vi "sv_Scale Factor for Change in Base Length Unit.vi"(5 "desired base units for length":i32(ring) items=["no change"=-1, "m"=0, "mm"=2, "microns"=3, "in"=1, "mils"=5], 7 "integration type":T1(ring), 8 "custom label in":string, 9 "engineering units in":T2 items=["custom..."=0, "V"=1, "A"=21, "C"=30, "pC"=31, "s"=32, "-"=29, "Pa"=2, "N"=20, "g"=3, "m/s^2"=4, "m/s"=5, "m"=6, "mm/s"=12, "mm"=13, "micron/s"=14, "micron"=15, "in/s^2"=7, "in/s"=8, "in"=9, "mil/s"=10, "mil"=11, "rad/s^2"=16, "rad/s"=17, "rad"=18, "deg/s^2"=26, "deg/s"=27, "deg"=28, "RPM"=22, "cycle/s^2"=23, "Hz"=24, "cycle"=25, "strain"=19], 10 "dB reference [EU] in":dbl) -> (0 "custom label out":string, 1 "engineering units out":T2 items=["custom..."=0, "V"=1, "A"=21, "C"=30, "pC"=31, "s"=32, "-"=29, "Pa"=2, "N"=20, "g"=3, "m/s^2"=4, "m/s"=5, "m"=6, "mm/s"=12, "mm"=13, "micron/s"=14, "micron"=15, "in/s^2"=7, "in/s"=8, "in"=9, "mil/s"=10, "mil"=11, "rad/s^2"=16, "rad/s"=17, "rad"=18, "deg/s^2"=26, "deg/s"=27, "deg"=28, "RPM"=22, "cycle/s^2"=23, "Hz"=24, "cycle"=25, "strain"=19], 2 "dB reference [EU] out":dbl, 3 "units scale factor":dbl)   [LabVIEW 2017]
uses:
  <vilib>/addons/_NISVFA/_Shared subVIs/Controls/svc_Engineering Units Text Ring.ctl
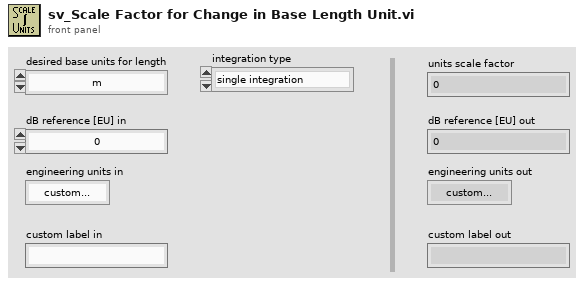
[diagram p1: front panel]
types:
  T1 = enum16{"single integration", "double integration"}
  T2 = typedef "svc_Engineering Units Text Ring.ctl" = u16
  T3 = enum16{"custom...", "V", "Pa", "g", "m/s^2", "m/s", "m", "in/s^2", "in/s", "in", "mil/s", "mil", "mm/s", "mm", "micron/s", "micron", "rad/s^2", "rad/s", "rad", "strain", "N", "A", "rpm", "cycle/s^2", "Hz", "cycle", "deg/s^2", "deg/s", "deg", "Undefined", "C", "pC"}
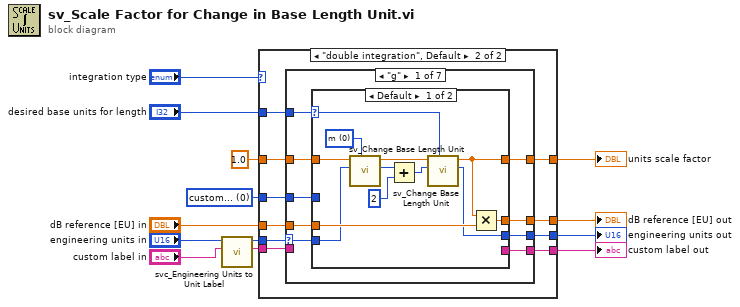
[diagram p0: block diagram]
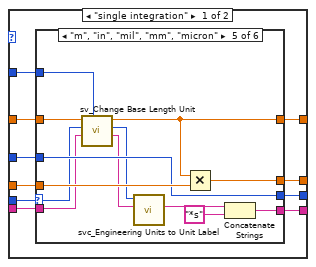
[diagram p2: hidden frame]
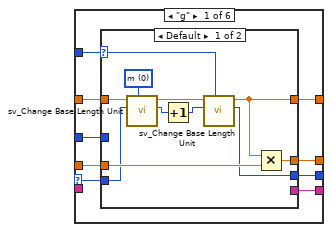
[diagram p3: hidden frame]
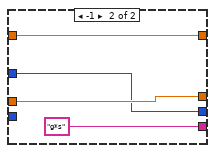
[diagram p4: hidden frame]
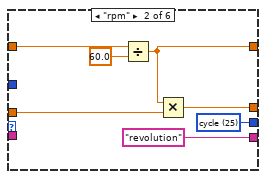
[diagram p5: hidden frame]
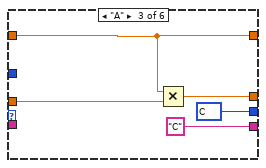
[diagram p6: hidden frame]
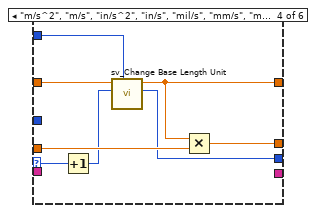
[diagram p7: hidden frame]
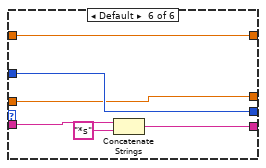
[diagram p8: hidden frame]
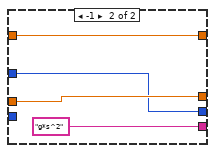
[diagram p9: hidden frame]
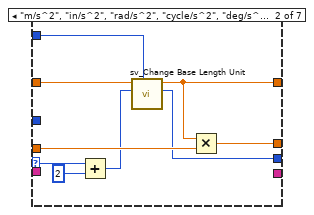
[diagram p10: hidden frame]
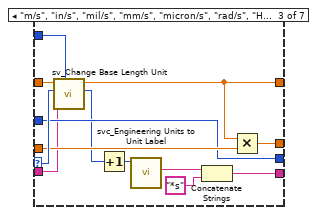
[diagram p11: hidden frame]
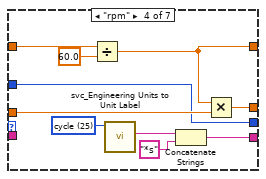
[diagram p12: hidden frame]
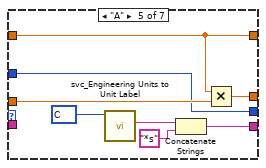
[diagram p13: hidden frame]
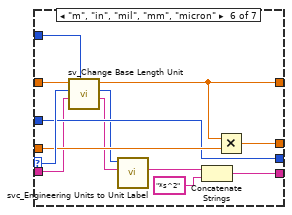
[diagram p14: hidden frame]
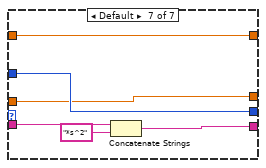
[diagram p15: hidden frame]
diagram:
  w10 = T2 0 items=["custom..."=0, "V"=1, "A"=21, "Pa"=2, "N"=20, "g"=3, "m/s^2"=4, "m/s"=5, "m"=6, "mm/s"=12, "mm"=13, "micron/s"=14, "micron"=15, "in/s^2"=7, "in/s"=8, "in"=9, "mil/s"=10, "mil"=11, "rad/s^2"=16, "rad/s"=17, "rad"=18, "m/m"=19] ("engineering units in")
  n1 = call <vilib>:"svc_Engineering Units to Unit Label.vi"("custom label"="custom label in", "engineering units"="engineering units in") -> ("unit label"=w8:string, "engineering units enum"=w2:T3)  [unwired: 8 in]
  n2 = case shown="\"double integration\", Default" "integration type" {
    tunnel: w2 -> [w23 w96]
    tunnel: [w22 w95] -> w6
    tunnel: 1.0 ("dB reference [EU]") -> [w21 w94]
    tunnel: "desired base units for length" -> [w19 w93]
    tunnel: "dB reference [EU] in" -> [w20 w92]
    tunnel: w8 -> [w18 w91]
    tunnel: [w17 w90] -> w9
    tunnel: [w16 w89] -> w11
    tunnel: [w14 w88] -> w12
    tunnel: w10 -> [w15 w87]
    frame "single integration" {
      n3 = case shown="\"m\", \"in\", \"mil\", \"mm\", \"micron\"" w23 {
        selector: w23 -> [w24 _ _ w62 w70 _]
        tunnel: [w31 w50 w55 w64 w77 w81] -> w22
        tunnel: w21 -> [w32 w54 w55 w67 w79 w81]
        tunnel: w20 -> [w30 w49 w57 w65 w76 w82]
        tunnel: w19 -> [w29 _ _ w66 w78 _]
        tunnel: w18 -> [_ _ _ _ w69 w85]
        tunnel: [w28 w48 w56 w63 w75 w82] -> w17
        tunnel: [w27 w52 w59 w60 w74 w84] -> w16
        tunnel: w15 -> [w25 _ _ _ w74 w84]
        tunnel: [w26 "revolution" ("Input Element") "C" ("Input Element") _ w73 w83] -> w14
        frame "g" {
          n4 = case shown="Default" w29 {
            selector: w29 -> [w35 _]
            tunnel: w32 -> [w39 w47]
            tunnel: [w34 w47] -> w31
            tunnel: w30 -> [w43 w46]
            tunnel: [w42 w46] -> w28
            tunnel: [w33 w44] -> w27
            tunnel: [_ "g*s" ("Input Element")] -> w26
            tunnel: w25 -> [_ w44]
            tunnel: w24 -> [w40 _]
            frame Default {
              w38 = 0 items=["no change"=-1, "m"=0, "mm"=2, "microns"=3, "in"=1, "mils"=5] ("desired base units for length")
              n5 = call <vilib>:"sv_Change Base Length Unit.vi"("desired base units for vibration"=w38, "engineering units in"=w40, "value in [EU]"=w39) -> ("engineering units out"=w41:T2, "value out [desired EU]"=w37:dbl)  [unwired: 4 in, 1 out]
              n6 = Increment(x=w41) -> (x+1=w36:T2)
              n7 = call <vilib>:"sv_Change Base Length Unit.vi"("desired base units for vibration"=w35, "engineering units in"=w36, "value in [EU]"=w37) -> ("engineering units out"=w33:T2, "value out [desired EU]"=w34:dbl)  [unwired: 4 in, 1 out]
              n8 = Multiply(x=w34, y=w43) -> (x*y=w42:dbl)
            }
            frame -1 {
            }
          }
        }
        frame "rpm" {
          w52 = T2 25 items=["custom..."=0, "V"=1, "A"=21, "Pa"=2, "N"=20, "g"=3, "m/s^2"=4, "m/s"=5, "m"=6, "mm/s"=12, "mm"=13, "micron/s"=14, "micron"=15, "in/s^2"=7, "in/s"=8, "in"=9, "mil/s"=10, "mil"=11, "rad/s^2"=16, "rad/s"=17, "rad"=18, "deg/s^2"=26, "deg/s"=27, "deg"=28, "RPM"=22, "cycle/s^2"=23, "Hz"=24, "cycle"=25, "strain"=19] ("engineering units in")
          n9 = Divide(x=w54, y=60.0) -> (x/y=w50:dbl)
          n10 = Multiply(x=w50, y=w49) -> (x*y=w48:dbl)
        }
        frame "A" {
          w59 = T2 30 items=["custom..."=0, "V"=1, "A"=21, "C"=30, "pC"=31, "s"=32, "-"=29, "Pa"=2, "N"=20, "g"=3, "m/s^2"=4, "m/s"=5, "m"=6, "mm/s"=12, "mm"=13, "micron/s"=14, "micron"=15, "in/s^2"=7, "in/s"=8, "in"=9, "mil/s"=10, "mil"=11, "rad/s^2"=16, "rad/s"=17, "rad"=18, "deg/s^2"=26, "deg/s"=27, "deg"=28, "RPM"=22, "cycle/s^2"=23, "Hz"=24, "cycle"=25, "strain"=19] ("engineering units in")
          n11 = Multiply(x=w55, y=w57) -> (x*y=w56:dbl)
        }
        frame "m/s^2", "m/s", "in/s^2", "in/s", "mil/s", "mm/s", "micron/s", "rad/s^2", "rad/s", "cycle/s^2", "Hz", "deg/s^2", "deg/s" {
          n12 = Increment(x=w62) -> (x+1=w61:T3)
          n13 = call <vilib>:"sv_Change Base Length Unit.vi"("desired base units for vibration"=w66, "engineering units in"=w61, "value in [EU]"=w67) -> ("engineering units out"=w60:T2, "value out [desired EU]"=w64:dbl)  [unwired: 4 in, 1 out]
          n14 = Multiply(x=w64, y=w65) -> (x*y=w63:dbl)
        }
        frame "m", "in", "mil", "mm", "micron" {
          n15 = call <vilib>:"sv_Change Base Length Unit.vi"("desired base units for vibration"=w78, "custom label in"=w69, "engineering units in"=w70, "value in [EU]"=w79) -> ("custom label out"=w68:string, "engineering units out"=w71:T2, "value out [desired EU]"=w77:dbl)  [unwired: 3 in]
          n16 = call <vilib>:"svc_Engineering Units to Unit Label.vi"("custom label"=w68, "engineering units"=w71) -> ("unit label"=w72:string)  [unwired: 8 in, 1 out]
          n17 = Multiply(x=w77, y=w76) -> (x*y=w75:dbl)
          n18 = Concatenate Strings(w72, "*s" ("Input Element")) -> (w73:string)
        }
        frame Default {
          n19 = Concatenate Strings(w85, "*s" ("Input Element")) -> (w83:string)
        }
      }
    }
    frame "double integration", Default {
      n20 = case shown="\"g\"" w96 {
        selector: w96 -> [w97 w124 w141 _ _ w172 _]
        tunnel: [w105 w129 w140 w145 w155 w171 w176] -> w95
        tunnel: w94 -> [w104 w130 w143 w147 w155 w174 w176]
        tunnel: w93 -> [w102 w127 w142 _ _ w173 _]
        tunnel: w92 -> [w103 w128 w139 w153 w161 w170 w175]
        tunnel: w91 -> [_ _ w131 _ _ w163 w179]
        tunnel: [w100 w126 w138 w152 w160 w169 w175] -> w90
        tunnel: [w101 w122 w137 w151 w159 w168 w177] -> w89
        tunnel: [w99 _ w136 w150 w158 w167 w178] -> w88
        tunnel: w87 -> [w98 _ w137 w151 w159 w168 w177]
        frame "g" {
          n21 = case shown="Default" w102 {
            selector: w102 -> [w115 _]
            tunnel: w104 -> [w109 w121]
            tunnel: [w116 w121] -> w105
            tunnel: w103 -> [w117 w120]
            tunnel: [w106 w118] -> w101
            tunnel: [w114 w120] -> w100
            tunnel: [_ "g*s^2" ("Input Element")] -> w99
            tunnel: w98 -> [_ w118]
            tunnel: w97 -> [w107 _]
            frame Default {
              w108 = 0 items=["no change"=-1, "m"=0, "mm"=2, "microns"=3, "in"=1, "mils"=5] ("desired base units for length")
              n22 = call <vilib>:"sv_Change Base Length Unit.vi"("desired base units for vibration"=w108, "engineering units in"=w107, "value in [EU]"=w109) -> ("engineering units out"=w112:T2, "value out [desired EU]"=w110:dbl)  [unwired: 4 in, 1 out]
              n23 = Add(x=w112, y=u16 2) -> (x+y=w111:T2)
              n24 = call <vilib>:"sv_Change Base Length Unit.vi"("desired base units for vibration"=w115, "engineering units in"=w111, "value in [EU]"=w110) -> ("engineering units out"=w106:T2, "value out [desired EU]"=w116:dbl)  [unwired: 4 in, 1 out]
              n25 = Multiply(x=w116, y=w117) -> (x*y=w114:dbl)
            }
            frame -1 {
            }
          }
        }
        frame "m/s^2", "in/s^2", "rad/s^2", "cycle/s^2", "deg/s^2" {
          n26 = Add(x=w124, y=u16 2) -> (x+y=w123:u16)
          n27 = call <vilib>:"sv_Change Base Length Unit.vi"("desired base units for vibration"=w127, "engineering units in"=w123, "value in [EU]"=w130) -> ("engineering units out"=w122:T2, "value out [desired EU]"=w129:dbl)  [unwired: 4 in, 1 out]
          n28 = Multiply(x=w129, y=w128) -> (x*y=w126:dbl)
        }
        frame "m/s", "in/s", "mil/s", "mm/s", "micron/s", "rad/s", "Hz", "deg/s" {
          n29 = call <vilib>:"sv_Change Base Length Unit.vi"("desired base units for vibration"=w142, "custom label in"=w131, "engineering units in"=w141, "value in [EU]"=w143) -> ("engineering units out"=w133:T2, "value out [desired EU]"=w140:dbl)  [unwired: 3 in, 1 out]
          n30 = Increment(x=w133) -> (x+1=w132:T2)
          n31 = call <vilib>:"svc_Engineering Units to Unit Label.vi"("engineering units"=w132) -> ("unit label"=w134:string)  [unwired: 9 in, 1 out]
          n32 = Concatenate Strings(w134, "*s" ("custom label")) -> (w136:string)
          n33 = Multiply(x=w140, y=w139) -> (x*y=w138:dbl)
        }
        frame "rpm" {
          w144 = T2 25 items=["custom..."=0, "V"=1, "A"=21, "Pa"=2, "N"=20, "g"=3, "m/s^2"=4, "m/s"=5, "m"=6, "mm/s"=12, "mm"=13, "micron/s"=14, "micron"=15, "in/s^2"=7, "in/s"=8, "in"=9, "mil/s"=10, "mil"=11, "rad/s^2"=16, "rad/s"=17, "rad"=18, "deg/s^2"=26, "deg/s"=27, "deg"=28, "RPM"=22, "cycle/s^2"=23, "Hz"=24, "cycle"=25, "strain"=19] ("engineering units")
          n34 = Divide(x=w147, y=60.0) -> (x/y=w145:dbl)
          n35 = call <vilib>:"svc_Engineering Units to Unit Label.vi"("engineering units"=w144) -> ("unit label"=w148:string)  [unwired: 9 in, 1 out]
          n36 = Concatenate Strings(w148, "*s" ("custom label")) -> (w150:string)
          n37 = Multiply(x=w145, y=w153) -> (x*y=w152:dbl)
        }
        frame "A" {
          w154 = T2 30 items=["custom..."=0, "V"=1, "A"=21, "C"=30, "pC"=31, "s"=32, "-"=29, "Pa"=2, "N"=20, "g"=3, "m/s^2"=4, "m/s"=5, "m"=6, "mm/s"=12, "mm"=13, "micron/s"=14, "micron"=15, "in/s^2"=7, "in/s"=8, "in"=9, "mil/s"=10, "mil"=11, "rad/s^2"=16, "rad/s"=17, "rad"=18, "deg/s^2"=26, "deg/s"=27, "deg"=28, "RPM"=22, "cycle/s^2"=23, "Hz"=24, "cycle"=25, "strain"=19] ("engineering units")
          n38 = call <vilib>:"svc_Engineering Units to Unit Label.vi"("engineering units"=w154) -> ("unit label"=w156:string)  [unwired: 9 in, 1 out]
          n39 = Concatenate Strings(w156, "*s" ("custom label")) -> (w158:string)
          n40 = Multiply(x=w155, y=w161) -> (x*y=w160:dbl)
        }
        frame "m", "in", "mil", "mm", "micron" {
          n41 = call <vilib>:"sv_Change Base Length Unit.vi"("desired base units for vibration"=w173, "custom label in"=w163, "engineering units in"=w172, "value in [EU]"=w174) -> ("custom label out"=w162:string, "engineering units out"=w164:T2, "value out [desired EU]"=w171:dbl)  [unwired: 3 in]
          n42 = call <vilib>:"svc_Engineering Units to Unit Label.vi"("custom label"=w162, "engineering units"=w164) -> ("unit label"=w165:string)  [unwired: 8 in, 1 out]
          n43 = Concatenate Strings(w165, "*s^2" ("custom label")) -> (w167:string)
          n44 = Multiply(x=w171, y=w170) -> (x*y=w169:dbl)
        }
        frame Default {
          n45 = Concatenate Strings(w179, "*s^2" ("Input Element")) -> (w178:string)
        }
      }
    }
  }
  "custom label out" <- w12
  "engineering units out" <- w11
  "dB reference [EU] out" <- w9
  "units scale factor" <- w6
